vi "Read ChnlNames.vi"(8 "error in (no error)":errorcluster, 11 "BME_DG_Base in":refnum<class "BME_DG_Base.lvclass">) -> (0 "error out":errorcluster, 2 "ChnlNames":string[](array[string]), 3 "BME_DG_Base out":refnum<class "BME_DG_Base.lvclass">)   [LabVIEW 2009, in "POLARIS BME DG.lvlib" / "BME_DG_Base.lvclass"]
uses:
  BME_DG_Base.lvclass
  BME_DG_Base.lvclass/BME_DG_Base.ctl
  BME_DG_Chnl/BME_DG_Chnl.lvclass
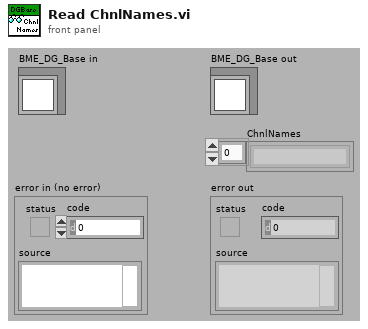
[diagram p1: front panel]
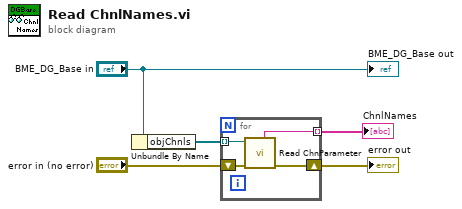
[diagram p0: block diagram]
diagram:
  n1 = Unbundle By Name("BME_DG_Base in") -> ("objChnls"=w2:refnum<class "BME_DG_Chnl.lvclass">[])
  n2 = for {
    tunnel: w2 -> [w9] mode=indexing
    tunnel: [w8] -> w1 mode=indexing
    shift-right: [w6] -> w4
    shift-left: "error in (no error)" -> [w7]
    n3 = call-dynamic "Read ChnParameter.vi"("error in (no error)"=w7, "BME_DG_Chnl in"=w9) -> ("error out"=w6:errorcluster, "Name"=w8:string)  [unwired: 4 in, 4 out]
  }
  "error out" <- w4
  "ChnlNames" <- w1
  "BME_DG_Base out" <- "BME_DG_Base in"
